vi "Determine_Save_Order.vi"(8 "error in (no error)":errorcluster, 10 "all VIs in memory":string[](array[string]), 11 "AB_Source in":refnum<class "AB_Source.lvclass">) -> (0 "error out":errorcluster, 2 "saveOrder":i32, 3 "AB_Source out":refnum<class "AB_Source.lvclass">)   [LabVIEW 2020, in "AB_Source.lvclass"]
uses:
  <vilib>/AppBuilder/AB_Classes/Source/AB_Source.lvclass
  <vilib>/Utility/lvfile.llb/NI_FileType.lvlib
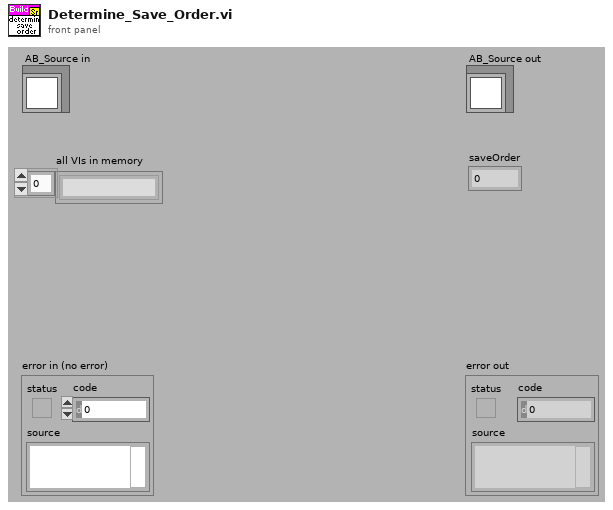
[diagram p1: front panel]
types:
  T1 = typedef "AB_Source.ctl" = cluster{"path":path, "itemID":string, "parentIndex":i32, "sourceInclusion":T2, "destinationIndex":i32, "properties":T3[], "newName":string, "lvfile":bool, "valid":bool, "eng_inBuild":bool, "eng_isNonVILink":bool, "Amalgamation":bool, "Amalgamation Piece":bool, "eng_delimitedName":string, "preventRename":bool}
  T2 = typedef "AB_Source_Inclusion.ctl" = enum16{"IncludeIfReferenced", "Include", "Exclude", "TopLevel"}
  T3 = typedef "AB_Source_Properties.ctl" = cluster{"sourcePropertyType":T4, "value":variant}
  T4 = typedef "AB_Source_Property_Type.ctl" = enum16{"Remove block diagram", "Remove front panel", "Password", "Window has title bar", "Show menu bar", "Show vertical scroll bar", "Show horizontal scroll bar", "Show toolbar", "Show Abort button", "Show fp when called", "Window behavior", "Allow user to close window", "Window run-time position", "Run when opened", "Allow debugging", "Auto error handling", "Generate guard code", "Use stack variables", "Expression folding", "Integer only", "Inline subVI"}
  T5 = typedef "NI_FileType.lvlib/FT_FileTypes.ctl" = enum32{"Invalid file/path", "Unknown type", "Instrument", "Control", "Polymorphic VI", "Project", "Library", "LVClass", "XControl", "XNode", "CIN", "Run-time menu", "Palette menu", "LLB", "Shortcut", "Directory", "Class Private Data Control", "Statechart", "MathScript .m file", "Ladder Diagram", "LVLibp"}
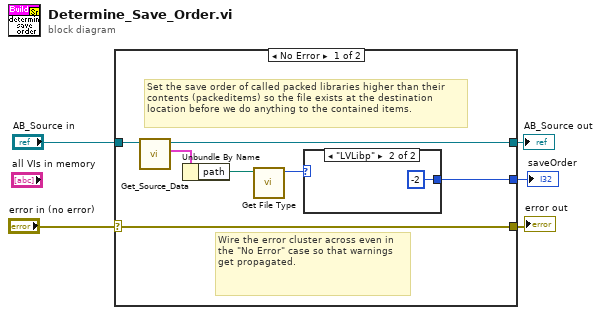
[diagram p0: block diagram]
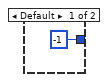
[diagram p2: hidden frame]
diagram:
  n1 = case shown="No Error" "error in (no error)" {
    selector: "error in (no error)" -> [w12 w16]
    tunnel: [w12 w16] -> w4
    tunnel: [w10 w15] -> w2
    tunnel: "AB_Source in" -> [w11 w15]
    tunnel: [w6 _] -> w1
    frame No Error {
      # "Set the save order of called packed libraries higher than their contents (packeditems) so the file exists at the destination location before we do anything to the contained items."
      # "Wire the error cluster across even in the \"No Error\" case so that warnings get propagated."
      n2 = call <vilib>:"Get_Source_Data.vi"("Class in"=w11) -> ("data"=w9:T1, "Class out"=w10:refnum<class "AB_Source.lvclass">)  [unwired: 8 in, 1 out]
      n3 = Unbundle By Name(w9) -> ("path"=w8:path)
      n4 = call <vilib>:"Get File Type.vi"("path"=w8) -> ("file type"=w7:T5)  [unwired: 8 in, 2 out]
      n5 = case shown="\"LVLibp\"" w7 {
        tunnel: [-1 -2] -> w6
        frame Default {
        }
        frame "LVLibp" {
        }
      }
    }
    frame Error {
    }
  }
  "error out" <- w4
  "AB_Source out" <- w2
  "saveOrder" <- w1
